vi "ReferenceMove.vi"(0 "object in":refnum<class "CetoniPump.lvclass">, 5 "error in (no error)":errorcluster) -> (14 "object out":refnum<class "CetoniPump.lvclass">, 19 "error out":errorcluster)   [LabVIEW 2024, in "CetoniPump.lvclass"]
uses:
  CetoniPump.lvclass
  CetoniPump.lvclass/CetoniPump.ctl
  Users/Lab user/AppData/Local/CETONI_SDK/lib/labview/labbCAN_Pump_API/labbCAN_Pump_API.lvlib
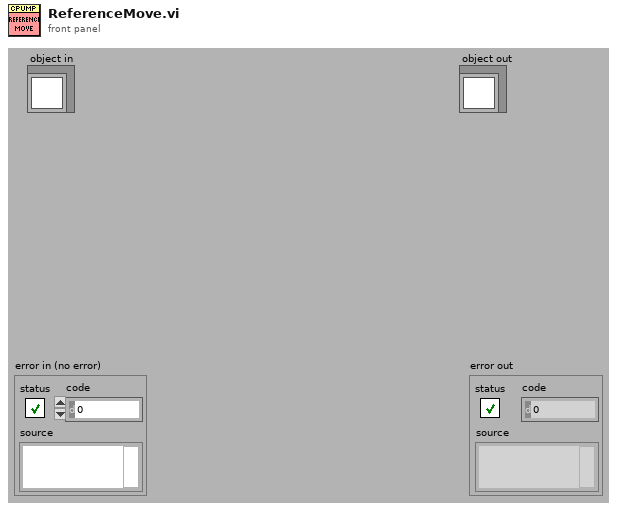
[diagram p1: front panel]
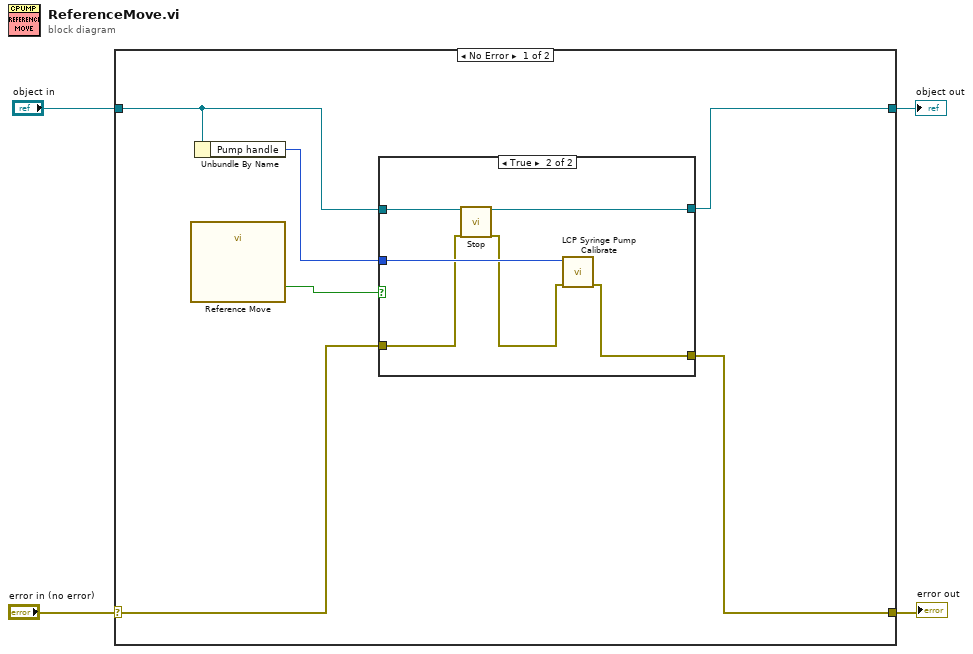
[diagram p0: block diagram]
diagram:
  n1 = case shown="No Error" "error in (no error)" {
    selector: "error in (no error)" -> [w9 w20]
    tunnel: [w8 w20] -> w3
    tunnel: [w6 w19] -> w1
    tunnel: "object in" -> [w5 w19]
    frame No Error {
      n2 = call "Reference Move"() -> ("OK"=w7:bool)  [unwired: 18 in, 1 out]
      n3 = Unbundle By Name(w5) -> ("Pump handle"=w10:i64)
      n4 = case shown="True" w7 {
        tunnel: w10 -> [_ w18]
        tunnel: w9 -> [w12 w14]
        tunnel: [w12 w17] -> w8
        tunnel: w5 -> [w11 w16]
        tunnel: [w11 w13] -> w6
        frame False {
        }
        frame True {
          n5 = call-dynamic "Stop.vi"("object in"=w16, "error in (no error)"=w14) -> ("object out"=w13:refnum<class "CetoniPump.lvclass">, "error out"=w15:errorcluster)  [unwired: 16 in]
          n6 = call "LCP Syringe Pump Calibrate.vi"("error in (no error)"=w15, "Pump Handle"=w18) -> ("error out"=w17:errorcluster)  [unwired: 9 in]
        }
      }
    }
    frame Error {
    }
  }
  "error out" <- w3
  "object out" <- w1
